vi "VerifPrevErrors.vi"(8 "error in (no error)":errorcluster, 11 "S4GUI in":refnum<class "S4GUI.lvclass">) -> (0 "error out":errorcluster, 3 "S4GUI out":refnum<class "S4GUI.lvclass">)   [LabVIEW 2018, in "S4GUI.lvclass"]
uses:
  S4GUI.lvclass
  S4GUI.lvclass/S4GUI.ctl
  Acquisition/Acquisition.lvclass
  Channel/Channel.lvclass
  StateMachine/State Machine.lvclass
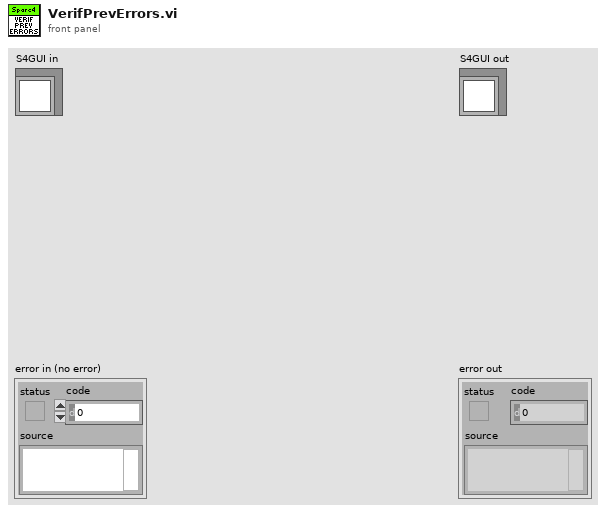
[diagram p1: front panel]
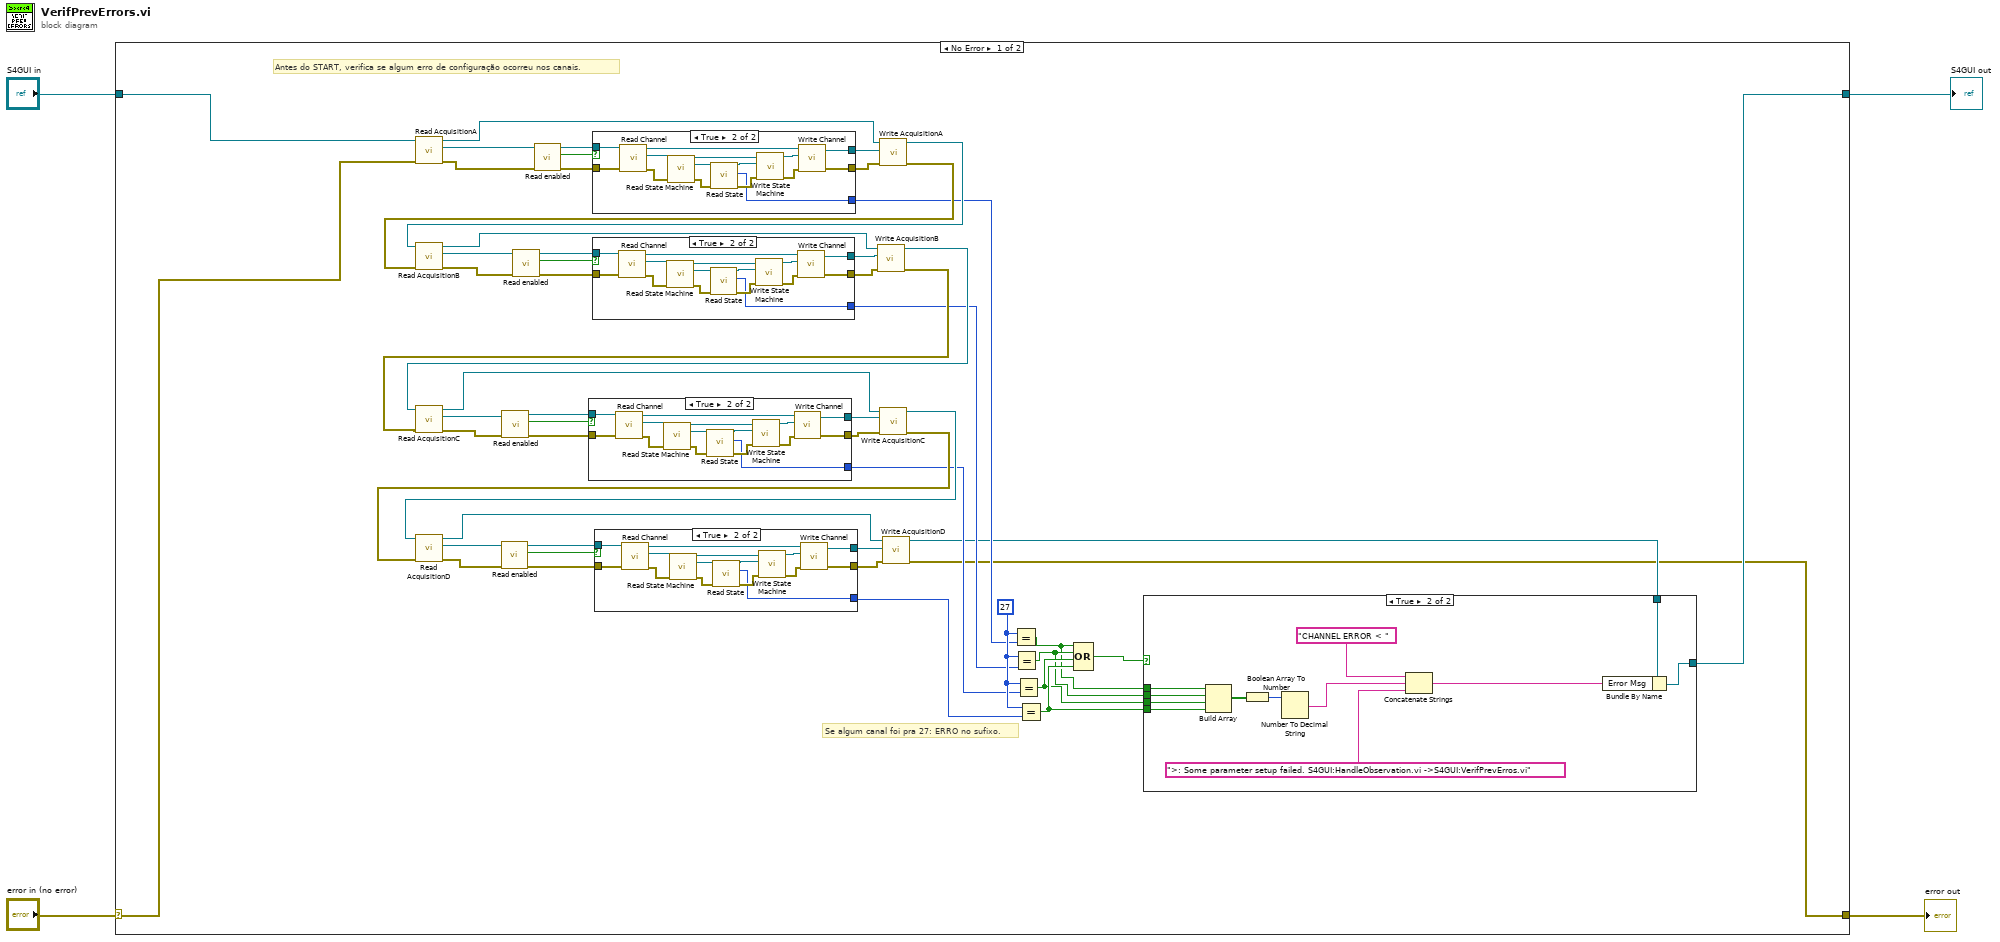
[diagram p0: block diagram]
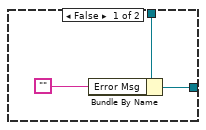
[diagram p2: hidden frame]
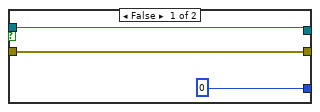
[diagram p3: hidden frame]
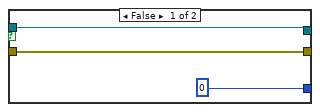
[diagram p4: hidden frame]
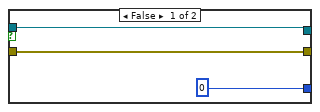
[diagram p5: hidden frame]
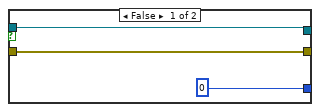
[diagram p6: hidden frame]
diagram:
  n1 = case shown="No Error" "error in (no error)" {
    selector: "error in (no error)" -> [w6 w146]
    tunnel: [w7 w146] -> w3
    tunnel: [w8 w145] -> w1
    tunnel: "S4GUI in" -> [w10 w145]
    frame No Error {
      w19 = 27 ("x")
      # "Antes do START, verifica se algum erro de configuração ocorreu nos canais."
      # "Se algum canal foi pra 27: ERRO no sufixo."
      n2 = call-dynamic "Read AcquisitionA.vi"("error in (no error)"=w6, "S4ACS_GUI in"=w10) -> ("error out"=w45:errorcluster, "Acquisition.lvclass"=w46:refnum<class "Acquisition.lvclass">, "S4ACS_GUI out"=w56:refnum<class "S4GUI.lvclass">)  [unwired: 7 in]
      n3 = call-dynamic "Read enabled.vi"("error in (no error)"=w45, "Server in"=w46) -> ("error out"=w43:errorcluster, "enabled"=w42:bool, "Server out"=w44:refnum<class "Acquisition.lvclass">)  [unwired: 7 in]
      n4 = case shown="True" w42 {
        tunnel: w44 -> [w128 w144]
        tunnel: w43 -> [w127 w143]
        tunnel: [w128 w141] -> w57
        tunnel: [w127 w140] -> w55
        tunnel: [0 ("State") w130] -> w18
        frame False {
        }
        frame True {
          n5 = call-dynamic "Read Channel.vi"("error in (no error)"=w143, "Acquisition in"=w144) -> ("error out"=w139:errorcluster, "Channel.lvclass"=w138:refnum<class "Channel.lvclass">, "Acquisition out"=w142:refnum<class "Acquisition.lvclass">)  [unwired: 7 in]
          n6 = call-dynamic "Read State Machine.vi"("error in (no error)"=w139, "Device in"=w138) -> ("error out"=w132:errorcluster, "State Machine.lvclass"=w134:refnum<class "State Machine.lvclass">, "Device out"=w136:refnum<class "Channel.lvclass">)  [unwired: 7 in]
          n7 = call-dynamic "Read State.vi"("error in (no error)"=w132, "State Machine in"=w134) -> ("error out"=w131:errorcluster, "State"=w130:i32, "State Machine out"=w133:refnum<class "State Machine.lvclass">)  [unwired: 7 in]
          n8 = call-dynamic "Write State Machine.vi"("error in (no error)"=w131, "State Machine.lvclass"=w133, "Device in"=w136) -> ("error out"=w135:errorcluster, "Device out"=w137:refnum<class "Channel.lvclass">)  [unwired: 7 in]
          n9 = call-dynamic "Write Channel.vi"("error in (no error)"=w135, "Channel.lvclass"=w137, "Acquisition in"=w142) -> ("error out"=w140:errorcluster, "Acquisition out"=w141:refnum<class "Acquisition.lvclass">)  [unwired: 7 in]
        }
      }
      n10 = call-dynamic "Write AcquisitionA.vi"("error in (no error)"=w55, "Acquisition.lvclass"=w57, "S4ACS_GUI in"=w56) -> ("error out"=w52:errorcluster, "S4ACS_GUI out"=w51:refnum<class "S4GUI.lvclass">)  [unwired: 7 in]
      n11 = call "Read AcquisitionB.vi"("error in (no error)"=w52, "S4ACS_GUI in"=w51) -> ("error out"=w37:errorcluster, "Acquisition.lvclass"=w40:refnum<class "Acquisition.lvclass">, "S4ACS_GUI out"=w41:refnum<class "S4GUI.lvclass">)  [unwired: 7 in]
      n12 = call-dynamic "Read enabled.vi"("error in (no error)"=w37, "Server in"=w40) -> ("error out"=w36:errorcluster, "enabled"=w38:bool, "Server out"=w39:refnum<class "Acquisition.lvclass">)  [unwired: 7 in]
      n13 = case shown="True" w38 {
        tunnel: w39 -> [w110 w126]
        tunnel: w36 -> [w109 w125]
        tunnel: [w110 w123] -> w35
        tunnel: [w109 w122] -> w34
        tunnel: [0 ("State") w112] -> w17
        frame False {
        }
        frame True {
          n14 = call-dynamic "Read Channel.vi"("error in (no error)"=w125, "Acquisition in"=w126) -> ("error out"=w121:errorcluster, "Channel.lvclass"=w120:refnum<class "Channel.lvclass">, "Acquisition out"=w124:refnum<class "Acquisition.lvclass">)  [unwired: 7 in]
          n15 = call-dynamic "Read State Machine.vi"("error in (no error)"=w121, "Device in"=w120) -> ("error out"=w114:errorcluster, "State Machine.lvclass"=w116:refnum<class "State Machine.lvclass">, "Device out"=w118:refnum<class "Channel.lvclass">)  [unwired: 7 in]
          n16 = call-dynamic "Read State.vi"("error in (no error)"=w114, "State Machine in"=w116) -> ("error out"=w113:errorcluster, "State"=w112:i32, "State Machine out"=w115:refnum<class "State Machine.lvclass">)  [unwired: 7 in]
          n17 = call-dynamic "Write State Machine.vi"("error in (no error)"=w113, "State Machine.lvclass"=w115, "Device in"=w118) -> ("error out"=w117:errorcluster, "Device out"=w119:refnum<class "Channel.lvclass">)  [unwired: 7 in]
          n18 = call-dynamic "Write Channel.vi"("error in (no error)"=w117, "Channel.lvclass"=w119, "Acquisition in"=w124) -> ("error out"=w122:errorcluster, "Acquisition out"=w123:refnum<class "Acquisition.lvclass">)  [unwired: 7 in]
        }
      }
      n19 = call "Write AcquisitionB.vi"("error in (no error)"=w34, "Acquisition.lvclass"=w35, "S4ACS_GUI in"=w41) -> ("error out"=w50:errorcluster, "S4ACS_GUI out"=w49:refnum<class "S4GUI.lvclass">)  [unwired: 7 in]
      n20 = call-dynamic "Read AcquisitionC.vi"("error in (no error)"=w50, "S4ACS_GUI in"=w49) -> ("error out"=w32:errorcluster, "Acquisition.lvclass"=w33:refnum<class "Acquisition.lvclass">, "S4ACS_GUI out"=w54:refnum<class "S4GUI.lvclass">)  [unwired: 7 in]
      n21 = call-dynamic "Read enabled.vi"("error in (no error)"=w32, "Server in"=w33) -> ("error out"=w31:errorcluster, "enabled"=w29:bool, "Server out"=w30:refnum<class "Acquisition.lvclass">)  [unwired: 7 in]
      n22 = case shown="True" w29 {
        tunnel: w30 -> [w92 w108]
        tunnel: w31 -> [w91 w107]
        tunnel: [w92 w105] -> w28
        tunnel: [w91 w104] -> w27
        tunnel: [0 ("State") w94] -> w16
        frame False {
        }
        frame True {
          n23 = call-dynamic "Read Channel.vi"("error in (no error)"=w107, "Acquisition in"=w108) -> ("error out"=w103:errorcluster, "Channel.lvclass"=w102:refnum<class "Channel.lvclass">, "Acquisition out"=w106:refnum<class "Acquisition.lvclass">)  [unwired: 7 in]
          n24 = call-dynamic "Read State Machine.vi"("error in (no error)"=w103, "Device in"=w102) -> ("error out"=w96:errorcluster, "State Machine.lvclass"=w98:refnum<class "State Machine.lvclass">, "Device out"=w100:refnum<class "Channel.lvclass">)  [unwired: 7 in]
          n25 = call-dynamic "Read State.vi"("error in (no error)"=w96, "State Machine in"=w98) -> ("error out"=w95:errorcluster, "State"=w94:i32, "State Machine out"=w97:refnum<class "State Machine.lvclass">)  [unwired: 7 in]
          n26 = call-dynamic "Write State Machine.vi"("error in (no error)"=w95, "State Machine.lvclass"=w97, "Device in"=w100) -> ("error out"=w99:errorcluster, "Device out"=w101:refnum<class "Channel.lvclass">)  [unwired: 7 in]
          n27 = call-dynamic "Write Channel.vi"("error in (no error)"=w99, "Channel.lvclass"=w101, "Acquisition in"=w106) -> ("error out"=w104:errorcluster, "Acquisition out"=w105:refnum<class "Acquisition.lvclass">)  [unwired: 7 in]
        }
      }
      n28 = call-dynamic "Write AcquisitionC.vi"("error in (no error)"=w27, "Acquisition.lvclass"=w28, "S4ACS_GUI in"=w54) -> ("error out"=w48:errorcluster, "S4ACS_GUI out"=w47:refnum<class "S4GUI.lvclass">)  [unwired: 7 in]
      n29 = call-dynamic "Read AcquisitionD.vi"("error in (no error)"=w48, "S4ACS_GUI in"=w47) -> ("error out"=w24:errorcluster, "Acquisition.lvclass"=w26:refnum<class "Acquisition.lvclass">, "S4ACS_GUI out"=w53:refnum<class "S4GUI.lvclass">)  [unwired: 7 in]
      n30 = call-dynamic "Read enabled.vi"("error in (no error)"=w24, "Server in"=w26) -> ("error out"=w23:errorcluster, "enabled"=w22:bool, "Server out"=w25:refnum<class "Acquisition.lvclass">)  [unwired: 7 in]
      n31 = case shown="True" w22 {
        tunnel: w25 -> [w74 w90]
        tunnel: w23 -> [w73 w89]
        tunnel: [w74 w87] -> w21
        tunnel: [w73 w86] -> w20
        tunnel: [0 ("State") w76] -> w15
        frame False {
        }
        frame True {
          n32 = call-dynamic "Read Channel.vi"("error in (no error)"=w89, "Acquisition in"=w90) -> ("error out"=w85:errorcluster, "Channel.lvclass"=w84:refnum<class "Channel.lvclass">, "Acquisition out"=w88:refnum<class "Acquisition.lvclass">)  [unwired: 7 in]
          n33 = call-dynamic "Read State Machine.vi"("error in (no error)"=w85, "Device in"=w84) -> ("error out"=w78:errorcluster, "State Machine.lvclass"=w80:refnum<class "State Machine.lvclass">, "Device out"=w82:refnum<class "Channel.lvclass">)  [unwired: 7 in]
          n34 = call-dynamic "Read State.vi"("error in (no error)"=w78, "State Machine in"=w80) -> ("error out"=w77:errorcluster, "State"=w76:i32, "State Machine out"=w79:refnum<class "State Machine.lvclass">)  [unwired: 7 in]
          n35 = call-dynamic "Write State Machine.vi"("error in (no error)"=w77, "State Machine.lvclass"=w79, "Device in"=w82) -> ("error out"=w81:errorcluster, "Device out"=w83:refnum<class "Channel.lvclass">)  [unwired: 7 in]
          n36 = call-dynamic "Write Channel.vi"("error in (no error)"=w81, "Channel.lvclass"=w83, "Acquisition in"=w88) -> ("error out"=w86:errorcluster, "Acquisition out"=w87:refnum<class "Acquisition.lvclass">)  [unwired: 7 in]
        }
      }
      n37 = call-dynamic "Write AcquisitionD.vi"("error in (no error)"=w20, "Acquisition.lvclass"=w21, "S4ACS_GUI in"=w53) -> ("error out"=w7:errorcluster, "S4ACS_GUI out"=w9:refnum<class "S4GUI.lvclass">)  [unwired: 7 in]
      n38 = Equal?(x=w19, y=w18) -> (x = y?=w11:bool)
      n39 = Equal?(x=w19, y=w17) -> (x = y?=w12:bool)
      n40 = Equal?(x=w19, y=w16) -> (x = y?=w13:bool)
      n41 = Equal?(x=w19, y=w15) -> (x = y?=w14:bool)
      n42 = Compound Arithmetic op=OR(w11, w12, w13, w14) -> (w5:bool)
      n43 = case shown="True" w5 {
        tunnel: w9 -> [w60 w72]
        tunnel: [w59 w71] -> w8
        tunnel: w14 -> [_ w65]
        tunnel: w13 -> [_ w66]
        tunnel: w12 -> [_ w67]
        tunnel: w11 -> [_ w68]
        frame False {
          n44 = Bundle By Name(cluster=w60, "Error Msg"="") -> (w59:refnum<class "S4GUI.lvclass">)
        }
        frame True {
          n45 = Build Array(w68, w67, w66, w65) -> (w70:bool[])
          n46 = Boolean Array To Number(Boolean array=w70) -> (number=w69:u32)
          n47 = Number To Decimal String(number=w69) -> (decimal integer string=w63:string)  [unwired: 1 in]
          n48 = Concatenate Strings("CHANNEL ERROR < " ("string"), w63, ">: Some parameter setup failed. S4GUI:HandleObservation.vi ->S4GUI:VerifPrevErros.vi" ("Error Msg")) -> (w62:string)
          n49 = Bundle By Name(cluster=w72, "Error Msg"=w62) -> (w71:refnum<class "S4GUI.lvclass">)
        }
      }
    }
    frame Error {
    }
  }
  "error out" <- w3
  "S4GUI out" <- w1
